vi "write_temp.vi"(1 "Temperature (C)":dbl) -> ()   [LabVIEW 2011]
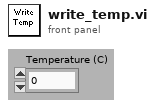
[diagram p1: front panel]
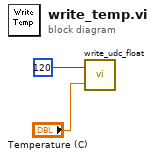
[diagram p0: block diagram]
diagram:
  n1 = call "write_udc_float.vi"("Value"="Temperature (C)", "Hex Address"=u16 120) -> ()  [unwired: 1 out]
